vi "power out sim.vi"(7 "Max Voltage in (V)":dbl=8.5 format="%.2f", 9 "Normalized Power (0-1)":dbl format="%.2f", 11 "error in (no error)":errorcluster) -> (8 "Max Voltage out (V)":dbl=8.5 format="%.2f", 15 "error out":errorcluster)   [LabVIEW 2016]
doc: "This one shot VI sets the power out using the thermal simulator\n\nPaul K Dixon\nPhysics 350\nCSUSB Physics"
uses:
  therm sim/therm sim kernel/globals/therm sim globals.vi
panel:
  in  "Clear":bool
  in  "Device":tag="Dev1"
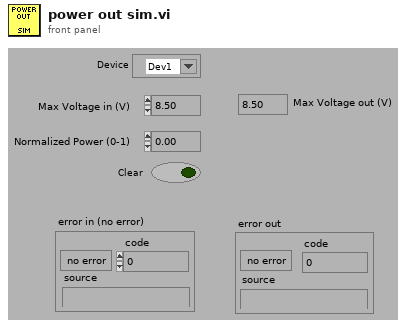
[diagram p1: front panel]
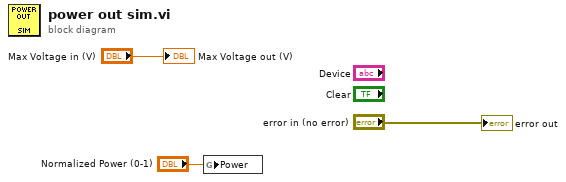
[diagram p0: block diagram]
diagram:
  n1 = global write "therm sim globals.vi" "Power"("Normalized Power (0-1)") -> ()
  "Max Voltage out (V)" <- "Max Voltage in (V)"
  "error out" <- "error in (no error)"
